vi "split memory hierarchy.vi"(8 "error in":errorcluster, 10 "UID":string, 11 "memory hierarchy":T1) -> (0 "error out":errorcluster, 2 "flat hierarchy with UID":T1, 3 "flat hierarchy without UID":T1)   [LabVIEW 2013, in "NISE_CEF_TreeSerializer.lvlib"]
uses:
  NISE_CEF_TreeSerializer.lvlib
  memory hierarchy.ctl
  full hierarchy.ctl
  hierarchy element.ctl
  serializable configuration/NISE_CEF_serializable configuration.lvclass
  serializable configuration/NISE_CEF_serializable configuration.lvclass/NISE_CEF_serializable configuration.ctl
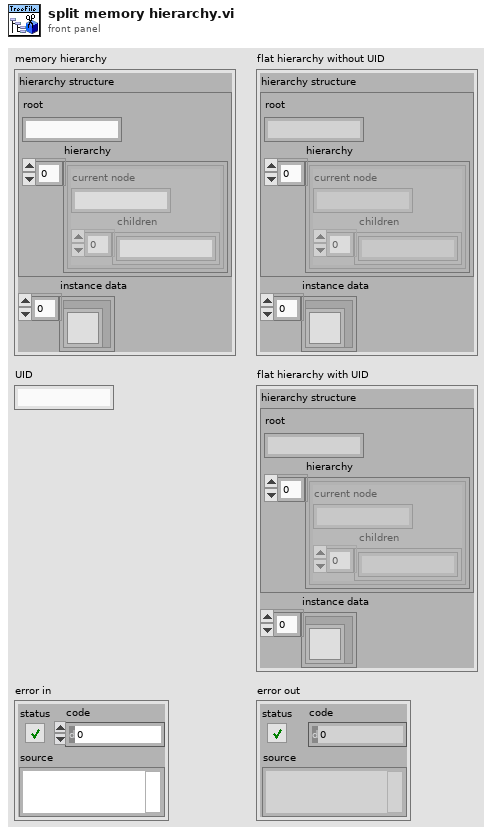
[diagram p1: front panel]
types:
  T1 = typedef "NISE_CEF_TreeSerializer.lvlib/memory hierarchy.ctl" = cluster{"hierarchy structure":T2, "instance data":refnum<class "NISE_CEF_serializable configuration.lvclass">[]}
  T2 = typedef "NISE_CEF_TreeSerializer.lvlib/full hierarchy.ctl" = cluster{"root":string, "hierarchy":T3[]}
  T3 = typedef "NISE_CEF_TreeSerializer.lvlib/hierarchy element.ctl" = cluster{"current node":string, "children":string[]}
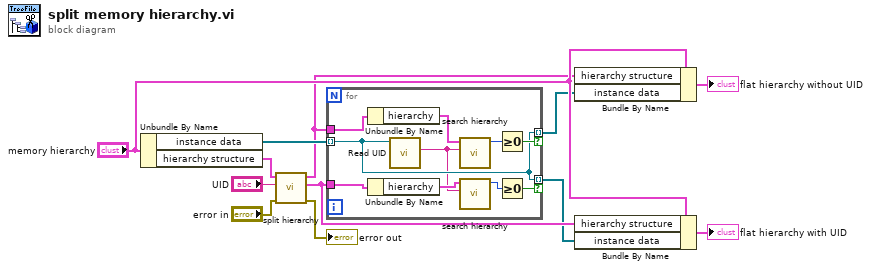
[diagram p0: block diagram]
diagram:
  n1 = Unbundle By Name("memory hierarchy") -> ("instance data"=w6:refnum<class "NISE_CEF_serializable configuration.lvclass">[], "hierarchy structure"=w12:T2)
  n2 = call "split hierarchy.vi"("error in"="error in", "UID to split"="UID", "hierarchy structure"=w12) -> ("error out"=→"error out":errorcluster, "hierarchy containing UID"=w4:T2, "hierarchy excluding UID"=w5:T2)  [unwired: 5 in, 1 out]
  n3 = for {
    tunnel: w6 -> [w14] mode=indexing
    tunnel: w5 -> [w22]
    tunnel: w4 -> [w21]
    tunnel: [w14] -> w2 mode=indexing if=w15
    tunnel: [w14] -> w3 mode=indexing if=w16
    n4 = Unbundle By Name(w22) -> ("hierarchy"=w19:T3[])
    n5 = Unbundle By Name(w21) -> ("hierarchy"=w20:T3[])
    n6 = call "Read UID.vi"("configuration in"=w14) -> ("instance id"=w13:string)  [unwired: 8 in, 2 out]
    n7 = call "search hierarchy.vi"("ID"=w13, "hierarchy"=w19) -> ("index"=w18:i32)  [unwired: 9 in]
    n8 = call "search hierarchy.vi"("ID"=w13, "hierarchy"=w20) -> ("index"=w17:i32)  [unwired: 9 in]
    n9 = Greater Or Equal To 0?(x=w18) -> (x >= 0?=w15:bool)
    n10 = Greater Or Equal To 0?(x=w17) -> (x >= 0?=w16:bool)
  }
  n11 = Bundle By Name(cluster="memory hierarchy", "hierarchy structure"=w5, "instance data"=w2) -> (→"flat hierarchy without UID":T1)
  n12 = Bundle By Name(cluster="memory hierarchy", "hierarchy structure"=w4, "instance data"=w3) -> (→"flat hierarchy with UID":T1)
